vi "Begin.vi"(8 "error in":errorcluster) -> (0 "error out":errorcluster)   [LabVIEW 2019]
doc: "Called before other user functions, this VI is expected to open initial I/O refnums, load in file data, and do all program initialization. Notice that the <B>error out</B> terminal is simply used for data flow. Wiring it to other structures or subVIs ensures that this VI runs first."
uses:
  <vilib>/Rock Robotics/SystemInterfaces/i2clib/i2c_bus.ctl
  <vilib>/Rock Robotics/WPI/DriverStation/WPI_DriverStationRobotMode2.ctl
  <vilib>/Rock Robotics/WPI/Joystick/WPI_JoystickDeviceEnum.ctl
  <vilib>/Rock Robotics/WPI/SafetyOutput/WPI_SafetyOutputConfigMenu.ctl
  <vilib>/Rock Robotics/WPI/ThirdParty/Phoenix-LabVIEW/Motor Controller/Controls/CTRE_Phoenix_MotorControl_ControlMode.ctl
  <vilib>/Rock Robotics/WPI/Solenoid/WPI_SolenoidChannel.ctl
  <vilib>/Rock Robotics/WPI/ThirdParty/Phoenix-LabVIEW/Motor Controller/Controls/CTRE_Phoenix_MotorControl_NeutralMode.ctl
  <vilib>/Rock Robotics/WPI/ThirdParty/Phoenix-LabVIEW/Motor Controller/Controls/CTRE_Phoenix_MotorControl_FeedbackDevice.ctl
  <vilib>/Rock Robotics/WPI/ThirdParty/REV Robotics/SPARK MAX/Typedef/Spark MAX Motor Type.ctl
  <vilib>/Rock Robotics/WPI/ThirdParty/Phoenix-LabVIEW/Motor Controller/Controls/CTRE_Phoenix_MotorControl_FeedbackDevice_TalonFX.ctl
  <vilib>/Rock Robotics/WPI/ThirdParty/Phoenix-LabVIEW/Motor Controller/Controls/CTRE_Phoenix_MotorControl_VelocityMeasurementPeriod.ctl
  <vilib>/Rock Robotics/SystemInterfaces/DIO/FPGA_DIOChannel.ctl
  Robot Global Data.vi
  <vilib>/Rock Robotics/Network Tables/NT Write String Array.vi
  <vilib>/Rock Robotics/WPI/Solenoid/WPI_SolenoidOpenDouble.vi
  <vilib>/Rock Robotics/WPI/RobotDrive/WPI_RobotDriveOpen4MotorWithExistingMotors.vi
panel:
  in  "Blue Calibration":cluster{"R":dbl, "G":dbl, "B":dbl}={"R"=0.143, "G"=0.427, "B"=0.429}
  in  "Green Calibration":cluster{"R":dbl, "G":dbl, "B":dbl}={"R"=0.197, "G"=0.561, "B"=0.24}
  in  "Red Calibration":cluster{"R":dbl, "G":dbl, "B":dbl}={"R"=0.561, "G"=0.323, "B"=0.114}
  in  "Yellow Calibration":cluster{"R":dbl, "G":dbl, "B":dbl}={"R"=0.361, "G"=0.524, "B"=0.113}
  in  "I2C Bus":T1
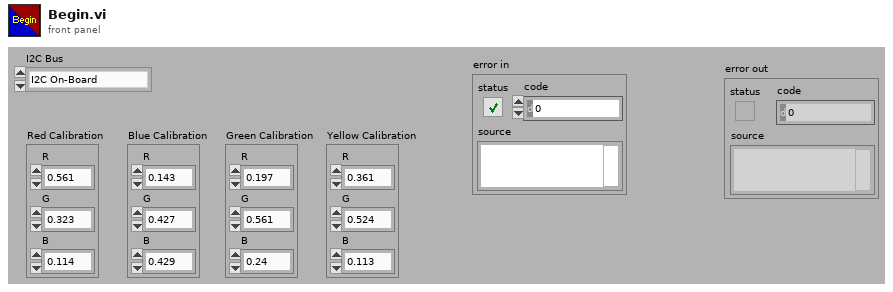
[diagram p1: front panel]
types:
  T1 = typedef "i2c_bus.ctl" = enum16{"I2C On-Board", "I2C MXP", "Invalid"}
  T2 = typedef "CTRE_Phoenix_MotorControl_NeutralMode.ctl" = enum8{"EEPROMSetting", "Override to Coast", "Override to Brake"}
  T3 = typedef "WPI_SolenoidChannel.ctl" = enum8{"Solenoid 0", "Solenoid 1", "Solenoid 2", "Solenoid 3", "Solenoid 4", "Solenoid 5", "Solenoid 6", "Solenoid 7", "Invalid"}
  T4 = typedef "FPGA_DIOChannel.ctl" = enum8{"DIO 0", "DIO 1", "DIO 2", "DIO 3", "DIO 4", "DIO 5", "DIO 6", "DIO 7", "DIO 8", "DIO 9", "DIO MXP 0", "DIO MXP 1", "DIO MXP 2", "DIO MXP 3", "DIO MXP 4", "DIO MXP 5", "DIO MXP 6", "DIO MXP 7", "DIO MXP 8", "DIO MXP 9", "DIO MXP 10", "DIO MXP 11", "DIO MXP 12", "DIO MXP 13", "DIO MXP 14", "DIO MXP 15", "SPI Port CS1", "SPI Port CS2", "SPI Port CS3", "SPI Port MISO", "SPI Port MOSI", "Invalid"}
  T5 = typedef "CTRE_Phoenix_MotorControl_VelocityMeasurementPeriod.ctl" = u16
  T6 = typedef "CTRE_Phoenix_MotorControl_FeedbackDevice_TalonFX.ctl" = i8
  T7 = typedef "CTRE_Phoenix_MotorControl_ControlMode.ctl" = u16
  T8 = typedef "Spark MAX Motor Type.ctl" = enum16{"Brushed", "Brushless"}
  T9 = typedef "CTRE_Phoenix_MotorControl_FeedbackDevice.ctl" = i8
  T10 = typedef "WPI_SafetyOutputConfigMenu.ctl" = enum16{"Enable", "Disable"}
  T11 = typedef "WPI_JoystickDeviceEnum.ctl" = enum16{"USB 0", "USB 1", "USB 2", "USB 3", "USB 4", "USB 5"}
  T12 = typedef "WPI_DriverStationRobotMode2.ctl" = enum16{"Autonomous Disabled", "Autonomous Enabled", "Teleop Disabled", "Teleop Enabled", "Disconnected", "Finish", "Test Disabled", "Test Enabled", "Emergency Stopped"}
  T13 = typedef "Color Sensor V3 DevRef.ctl" = cluster{"I2CDevRef":T14}
  T14 = typedef "WPI_I2CDevRef.ctl" = cluster{"DevStatus":errorcluster, "Device Address":u8, "Handle":i32, "I2C Bus":T1}
  T15 = typedef "WPI_JoystickDevRef.ctl" = cluster{"Device":T11}
  T16 = typedef "WPI_DigitalInputDevRef.ctl" = cluster{"DevStatus":errorcluster, "DIO Channel":T4}
  T17 = typedef "WPI_MotorControlDeviceRef.ctl" = cluster{"DeviceStatus":errorcluster, "Type":T18, "PWM":cluster{"PWM Channel":T19, "DeadBand":T20}, "CAN":cluster{"Device Number":u8, "SetOutput VI Ref":variant, "GetOutput VI Ref":variant, "Enable VI Ref":variant, "Disable VI Ref":variant, "Data":variant}, "Invert":bool, "DIO PWM":cluster{"PWM \"Enable\" Channel":T19, "DIOChannel":T4, "PWM Rate":dbl}}
  T18 = typedef "WPI_MotorControlType.ctl" = enum16{"PWM", "CAN", "DIO PWM"}
  T19 = typedef "FPGA_DIOPWMChannel.ctl" = enum8{"PWM 0", "PWM 1", "PWM 2", "PWM 3", "PWM 4", "PWM 5", "PWM 6", "PWM 7", "PWM 8", "PWM 9", "PWM MXP 0", "PWM MXP 1", "PWM MXP 2", "PWM MXP 3", "PWM MXP 4", "PWM MXP 5", "PWM MXP 6", "PWM MXP 7", "PWM MXP 8", "PWM MXP 9", "Invalid"}
  T20 = typedef "WPI_PWMDeadband.ctl" = cluster{"Name":string, "maxPositivePwm":i32, "minPositivePwm":i32, "centerPwm":i32, "maxNegativePwm":i32, "minNegativePwm":i32, "angularRange":u16}
  T21 = typedef "WPI_SolenoidDevRef.ctl" = cluster{"DevStatus":errorcluster, "Pneumatics Control Module":u8, "Forward Solenoid Channel":T3, "Reverse Solenoid Channel":T3}
  T22 = typedef "WPI_RobotDriveDevRef.ctl" = cluster{"DevStatus":errorcluster, "Motors[]":T17[], "Square Inputs":bool, "Max Output":dbl}
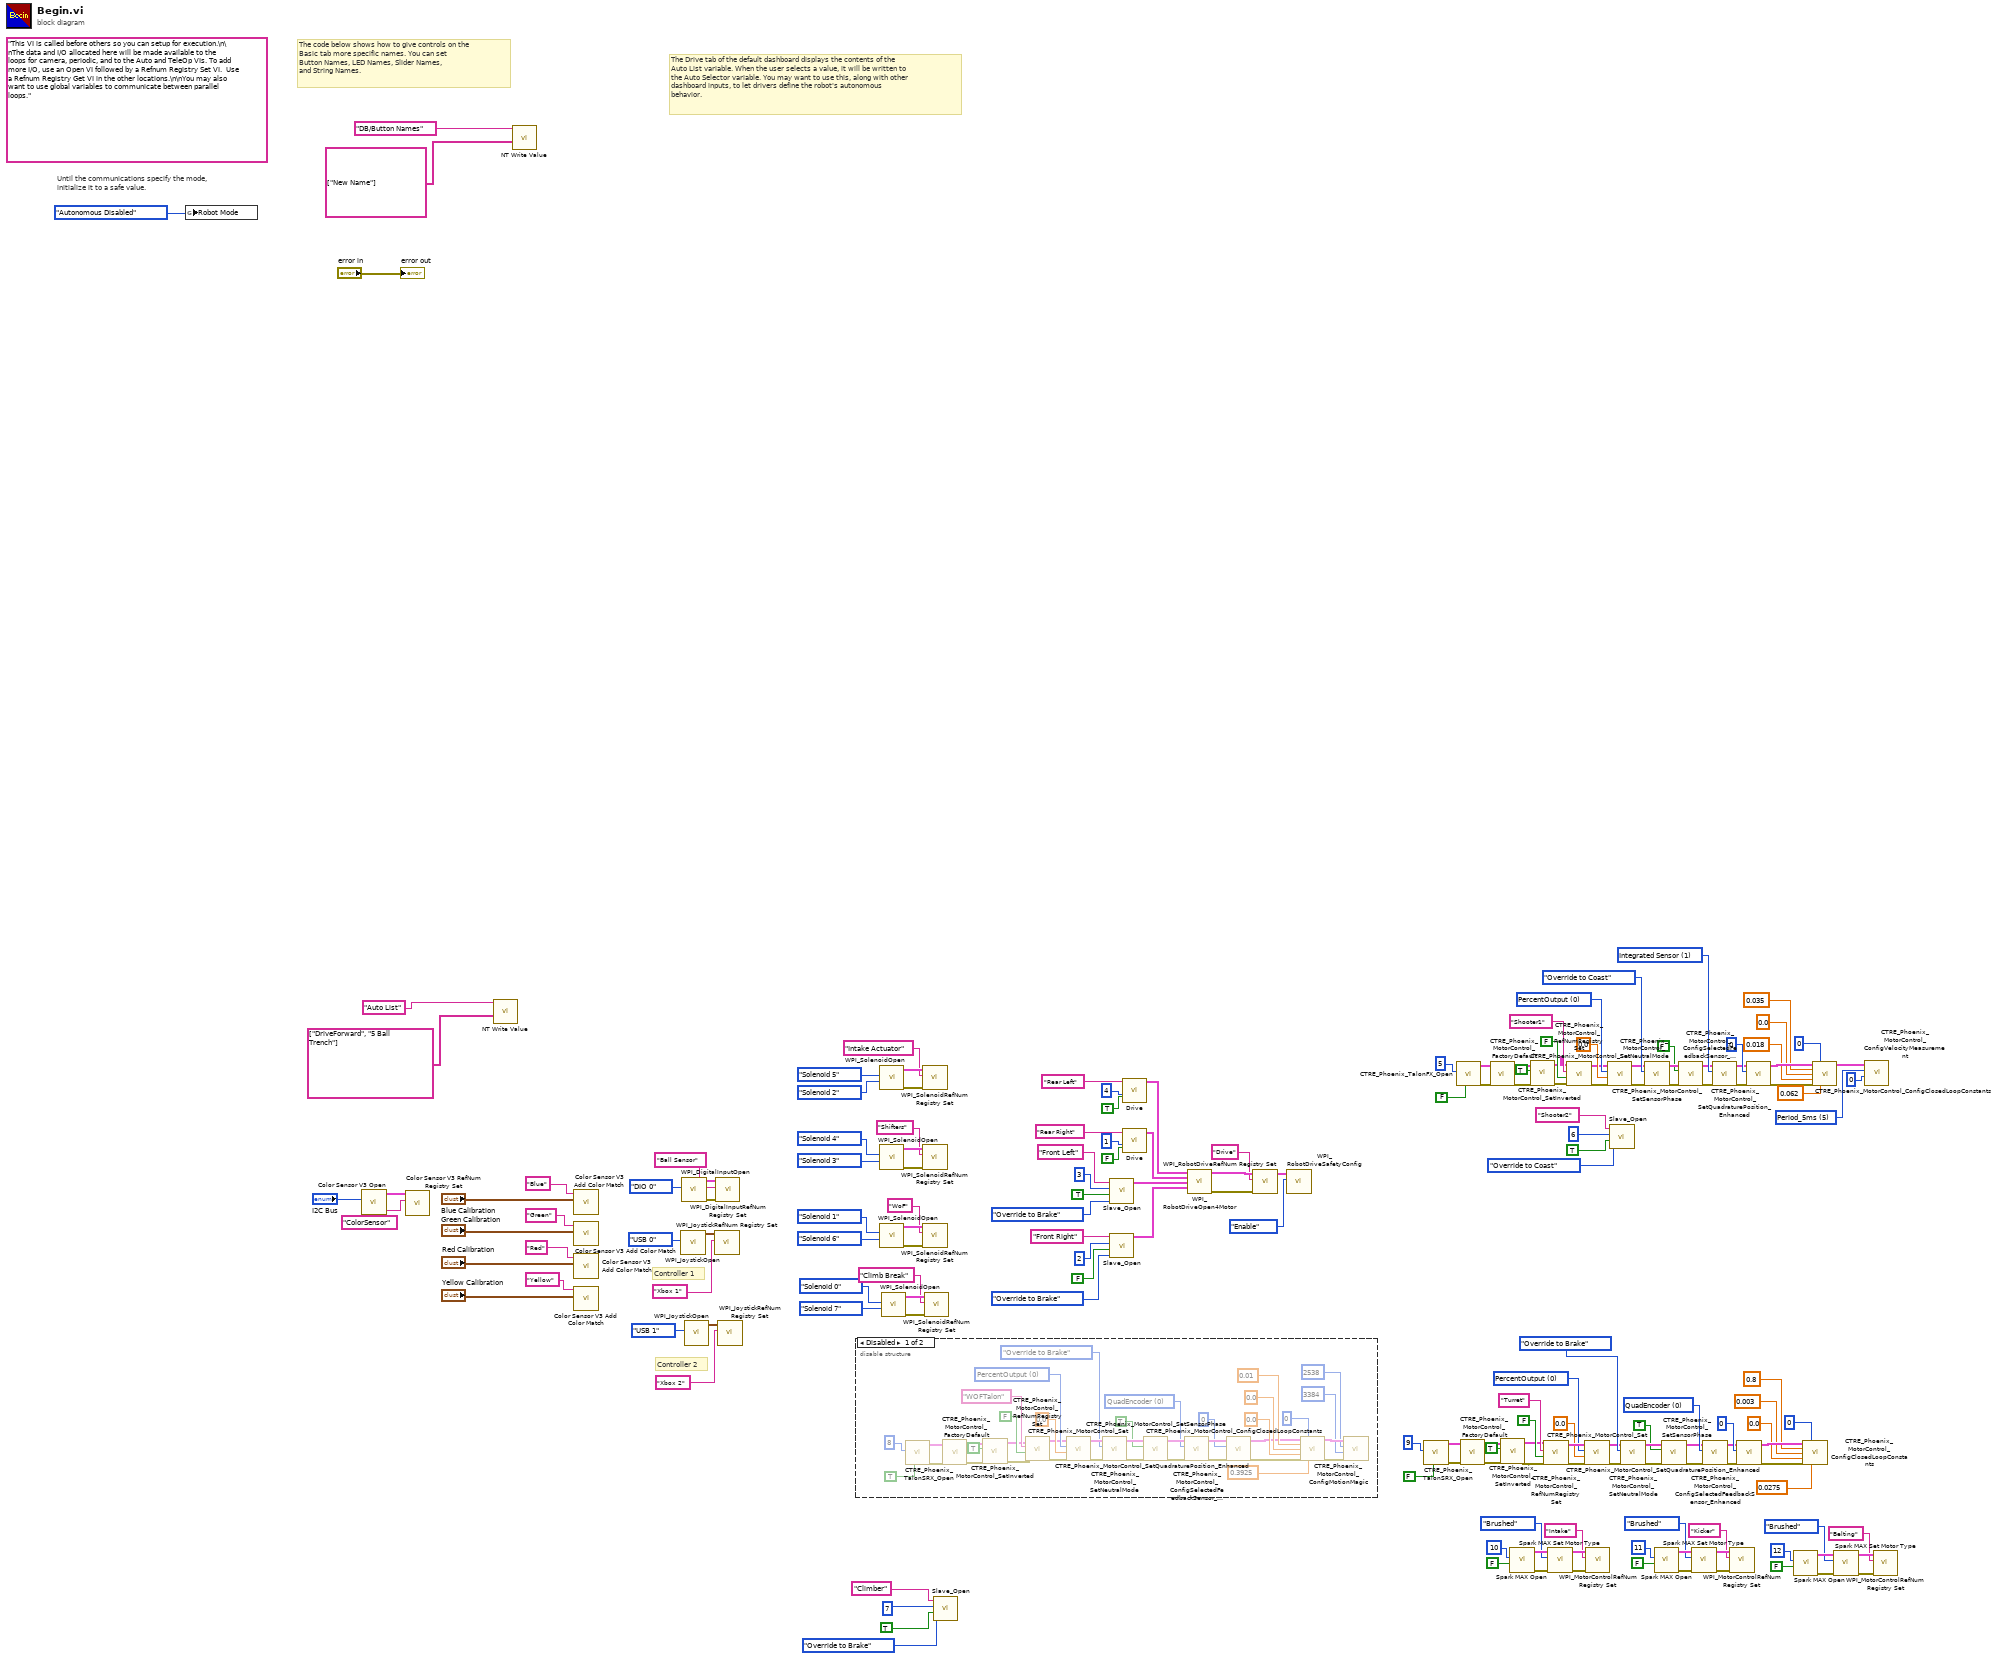
[diagram p0: block diagram]
diagram:
  w88 = T5 5 items=["Period_1ms"=1, "Period_2ms"=2, "Period_5ms"=5, "Period_10ms"=10, "Period_20ms"=20, "Period_25ms"=25, "Period_50ms"=50, "Period_100ms"=100] ("Velocity Measurement Period")
  w78 = T6 1 items=["Integrated Sensor"=1, "Sensor Sum (S0 + S1)"=9, "Sensor Difference (D0 - D1)"=10, "Remote Source 0"=11, "Remote Source 1"=12, "None"=14, "Software Emulated"=15] ("Talon FX Feedback Device")
  w76 = T7 0 items=["PercentOutput"=0, "Position"=1, "Velocity"=2, "Current"=3, "Follower"=5, "MotionProfile"=6, "MotionMagic"=7, "MotionProfileArc"=10, "Disabled"=15] ("Control Mode")
  w131 = T9 0 items=["None"=-1, "QuadEncoder"=0, "Analog"=2, "Tachometer"=4, "Pulse Width Encoded Position"=8, "Sensor Sum (S0 + S1)"=9, "Sensor Difference (D0 - D1)"=10, "Remote Source 0"=11, "Remote Source 1"=12, "Software Emulated"=15] ("Feedback Device")
  w136 = T7 0 items=["PercentOutput"=0, "Position"=1, "Velocity"=2, "Current"=3, "Follower"=5, "MotionProfile"=6, "MotionMagic"=7, "MotionMagicArc"=8, "MotionProfileArc"=10, "Disabled"=15] ("Control Mode")
  (unwired) "This VI is called before others so you can setup for execution.\n\nThe data and I/O allocated here will be made available to the loops for camera, periodic, and to the Auto and TeleOp VIs. To add more I/O, use an Open VI followed by a Refnum Registry Set VI.  Use a Refnum Registry Get VI in the other locations.\n\nYou may also want to use global variables to communicate between parallel loops."
  # "Controller 2"
  # "Controller 1"
  # "The Drive tab of the default dashboard displays the contents of the\nAuto List variable. When the user selects a value, it will be written to\nthe Auto Selector variable. You may want to use this, along with other\ndashboard inputs, to let drivers define the robot's autonomous\nbehavior."
  # "The code below shows how to give controls on the\nBasic tab more specific names. You can set\nButton Names, LED Names, Slider Names,\nand String Names."
  # "Until the communications specify the mode,\ninitialize it to a safe value."
  n1 = global write "Robot Global Data.vi" "Robot Mode"(WPI_DriverStationRobotMode2."Autonomous Disabled" ("Robot Mode")) -> ()
  n2 = call <vilib>:"Color Sensor V3 Open.vi"("I2C Bus"="I2C Bus") -> ("ColorSensorDevRef"=w155:T13)  [unwired: 9 in, 1 out]
  n3 = call <vilib>:"Color Sensor V3 RefNum Registry Set.vi"("refnum name"="ColorSensor", "ColorSensorDevRef"=w155) -> ()  [unwired: 8 in, 2 out]
  n4 = call-poly <vilib>:"NT Write Value.vi"("String Array"=string[] ["DriveForward", "5 Ball Trench"], "Name"="Auto List") -> ()  [unwired: 9 in, 1 out]
  n5 = call-poly <vilib>:"NT Write Value.vi"("String Array"=string[] ["New Name"], "Name"="DB/Button Names") -> ()  [unwired: 9 in, 1 out]
  n6 = call <vilib>:"Color Sensor V3 Add Color Match.vi"("Color"="Blue Calibration", "Name"="Blue") -> ()  [unwired: 10 in]
  n7 = call <vilib>:"Color Sensor V3 Add Color Match.vi"("Color"="Green Calibration", "Name"="Green") -> ()  [unwired: 10 in]
  n8 = call <vilib>:"Color Sensor V3 Add Color Match.vi"("Color"="Red Calibration", "Name"="Red") -> ()  [unwired: 10 in]
  n9 = call <vilib>:"Color Sensor V3 Add Color Match.vi"("Color"="Yellow Calibration", "Name"="Yellow") -> ()  [unwired: 10 in]
  n10 = call <vilib>:"WPI_JoystickOpen.vi"("JoystickDevice"=WPI_JoystickDeviceEnum."USB 0") -> ("JoystickDevRef"=w171:T15)  [unwired: 10 in]
  n11 = call <vilib>:"WPI_DigitalInputOpen.vi"("DIO Channel"=FPGA_DIOChannel."DIO 0") -> ("error out"=w59:errorcluster, "DigitalInputDevRef"=w58:T16)  [unwired: 9 in]
  n12 = call <vilib>:"WPI_JoystickOpen.vi"("JoystickDevice"=WPI_JoystickDeviceEnum."USB 1") -> ("JoystickDevRef"=w152:T15)  [unwired: 10 in]
  n13 = call <vilib>:"WPI_JoystickRefNum Registry Set.vi"("refnum name"="Xbox 1", "JoystickDevRef"=w171) -> ()  [unwired: 8 in, 2 out]
  n14 = call <vilib>:"WPI_DigitalInputRefNum Registry Set.vi"("error in (no error)"=w59, "refnum name"="Ball Sensor", "DigitalInputDevRef"=w58) -> ()  [unwired: 7 in, 2 out]
  n15 = call <vilib>:"WPI_JoystickRefNum Registry Set.vi"("refnum name"="Xbox 2", "JoystickDevRef"=w152) -> ()  [unwired: 8 in, 2 out]
  n16 = disable-structure shown="Disabled" {
    frame Disabled {
      w200 = T9 0 items=["None"=-1, "QuadEncoder"=0, "Analog"=2, "Tachometer"=4, "Pulse Width Encoded Position"=8, "Sensor Sum (S0 + S1)"=9, "Sensor Difference (D0 - D1)"=10, "Remote Source 0"=11, "Remote Source 1"=12, "Software Emulated"=15] ("Feedback Device")
      w195 = T7 0 items=["PercentOutput"=0, "Position"=1, "Velocity"=2, "Current"=3, "Follower"=5, "MotionProfile"=6, "MotionMagic"=7, "MotionMagicArc"=8, "MotionProfileArc"=10, "Disabled"=15] ("Control Mode")
      n17 = call <vilib>:"CTRE_Phoenix_TalonSRX_Open.vi"("Invert"=TRUE, "Device Number"=u8 8) -> ("error out"=w179:errorcluster, "CAN Talon SRX Ref"=w180:T17)  [unwired: 8 in]
      n18 = call <vilib>:"CTRE_Phoenix_MotorControl_FactoryDefault.vi"("error in"=w179, "PhoenixMotorControlDevRef"=w180) -> ("error out"=w178:errorcluster, "PhoenixMotorControlDevRef"=w177:T17)  [unwired: 8 in]
      n19 = call <vilib>:"CTRE_Phoenix_MotorControl_SetInverted.vi"("error in (no error)"=w178, "Invert?"=TRUE, "PhoenixMotorControlDevRef"=w177) -> ("error out"=w174:errorcluster, "PhoenixMotorControlDevRef"=w175:T17)  [unwired: 7 in]
      n20 = call <vilib>:"CTRE_Phoenix_MotorControl_RefNumRegistrySet.vi"("error in (no error)"=w174, "Test Mode Only"=FALSE, "refnum name"="WOFTalon", "PhoenixMotorControlDevRef"=w175) -> ("error out"=w193:errorcluster, "PhoenixMotorControlDevRef"=w194:T17)  [unwired: 6 in]
      n21 = call <vilib>:"CTRE_Phoenix_MotorControl_Set.vi"("error in (no error)"=w193, "Output"=0.0, "Control Mode"=w195, "PhoenixMotorControlDevRef"=w194) -> ("error out"=w204:errorcluster, "PhoenixMotorControlDevRef"=w208:T17)  [unwired: 6 in]
      n22 = call <vilib>:"CTRE_Phoenix_MotorControl_SetNeutralMode.vi"("error in (no error)"=w204, "Motor Control Neutral Mode"=CTRE_Phoenix_MotorControl_NeutralMode."Override to Brake", "PhoenixMotorControlDevRef"=w208) -> ("error out"=w206:errorcluster, "PhoenixMotorControlDevRef"=w205:T17)  [unwired: 7 in]
      n23 = call <vilib>:"CTRE_Phoenix_MotorControl_SetSensorPhase.vi"("error in (no error)"=w206, "PhaseSensor"=TRUE, "PhoenixMotorControlDevRef"=w205) -> ("error out"=w202:errorcluster, "PhoenixMotorControlDevRef"=w201:T17)  [unwired: 7 in]
      n24 = call <vilib>:"CTRE_Phoenix_MotorControl_ConfigSelectedFeedbackSensor_Enhanced.vi"("error in (no error)"=w202, "Feedback Device"=w200, "PhoenixMotorControlDevRef"=w201) -> ("error out"=w198:errorcluster, "PhoenixMotorControlDevRef"=w199:T17)  [unwired: 7 in]
      n25 = call <vilib>:"CTRE_Phoenix_MotorControl_SetQuadraturePosition_Enhanced.vi"("error in (no error)"=w198, "New Position"=0, "PhoenixMotorControlDevRef"=w199) -> ("error out"=w181:errorcluster, "PhoenixMotorControlDevRef"=w182:T17)  [unwired: 7 in]
      n26 = call <vilib>:"CTRE_Phoenix_MotorControl_ConfigClosedLoopConstants.vi"("PhoenixMotorControlDevRef"=w182, "slotIdx"=0, "P"=0.01, "I"=0.0, "D"=0.0, "error in (no error)"=w181, "F"=0.3925) -> ("PhoenixMotorControlDevRef"=w190:T17, "error out"=w191:errorcluster)  [unwired: 7 in]
      n27 = call <vilib>:"CTRE_Phoenix_MotorControl_ConfigMotionMagic.vi"("error in (no error)"=w191, "Acceleration"=3384, "Cruise Velocity"=2538, "PhoenixMotorControlDevRef"=w190) -> ()  [unwired: 6 in, 2 out]
    }
    frame Enabled {
    }
  }
  n28 = call-poly <vilib>:"WPI_SolenoidOpen.vi"("Reverse Solenoid Channel"=WPI_SolenoidChannel."Solenoid 2", "Forward Solenoid Channel"=WPI_SolenoidChannel."Solenoid 5") -> ("error out"=w46:errorcluster, "SolenoidDevRef"=w45:T21)  [unwired: 8 in]
  n29 = call-poly <vilib>:"WPI_SolenoidOpen.vi"("Reverse Solenoid Channel"=WPI_SolenoidChannel."Solenoid 3", "Forward Solenoid Channel"=WPI_SolenoidChannel."Solenoid 4") -> ("error out"=w117:errorcluster, "SolenoidDevRef"=w116:T21)  [unwired: 8 in]
  n30 = call-poly <vilib>:"WPI_SolenoidOpen.vi"("Reverse Solenoid Channel"=WPI_SolenoidChannel."Solenoid 6", "Forward Solenoid Channel"=WPI_SolenoidChannel."Solenoid 1") -> ("error out"=w55:errorcluster, "SolenoidDevRef"=w54:T21)  [unwired: 8 in]
  n31 = call-poly <vilib>:"WPI_SolenoidOpen.vi"("Reverse Solenoid Channel"=WPI_SolenoidChannel."Solenoid 7", "Forward Solenoid Channel"=WPI_SolenoidChannel."Solenoid 0") -> ("error out"=w51:errorcluster, "SolenoidDevRef"=w50:T21)  [unwired: 8 in]
  n32 = call <vilib>:"WPI_SolenoidRefNum Registry Set.vi"("error in (no error)"=w46, "refnum name"="Intake Actuator", "SolenoidDevRef"=w45) -> ()  [unwired: 7 in, 2 out]
  n33 = call <vilib>:"WPI_SolenoidRefNum Registry Set.vi"("error in (no error)"=w117, "refnum name"="Shifters", "SolenoidDevRef"=w116) -> ()  [unwired: 7 in, 2 out]
  n34 = call <vilib>:"WPI_SolenoidRefNum Registry Set.vi"("error in (no error)"=w55, "refnum name"="WoF", "SolenoidDevRef"=w54) -> ()  [unwired: 7 in, 2 out]
  n35 = call <vilib>:"WPI_SolenoidRefNum Registry Set.vi"("error in (no error)"=w51, "refnum name"="Climb Break", "SolenoidDevRef"=w50) -> ()  [unwired: 7 in, 2 out]
  n36 = call "Slave_Open.vi"("Motor Control Neutral Mode"=CTRE_Phoenix_MotorControl_NeutralMode."Override to Brake", "Invert"=TRUE, "Device Number"=u8 7, "Motor Name"="Climber" ("refnum name")) -> ()  [unwired: 7 in, 1 out]
  n37 = call "Slave_Open.vi"("Motor Control Neutral Mode"=CTRE_Phoenix_MotorControl_NeutralMode."Override to Brake", "Invert"=TRUE, "Device Number"=u8 3, "Motor Name"="Front Left" ("refnum name")) -> ("PhoenixMotorControlDevRef"=w12:T17)  [unwired: 7 in]
  n38 = call "Slave_Open.vi"("Motor Control Neutral Mode"=CTRE_Phoenix_MotorControl_NeutralMode."Override to Brake", "Invert"=FALSE, "Device Number"=u8 2, "Motor Name"="Front Right" ("refnum name")) -> ("PhoenixMotorControlDevRef"=w11:T17)  [unwired: 7 in]
  n39 = call "Drive.vi"("Invert"=TRUE, "Device Number"=u8 4, "Motor Name"="Rear Left" ("refnum name")) -> ("Motor Out"=w118:T17)  [unwired: 8 in]
  n40 = call "Drive.vi"("Invert"=FALSE, "Device Number"=u8 1, "Motor Name"="Rear Right" ("refnum name")) -> ("Motor Out"=w33:T17)  [unwired: 8 in]
  n41 = call-poly <vilib>:"WPI_RobotDriveOpen4Motor.vi"("Rear Left Motor Dev Ref"=w118, "Rear Right Motor Dev Ref"=w33, "Front Left Motor Dev Ref"=w12, "Front Right Motor Dev Ref"=w11) -> ("RobotDriveDevRef"=w150:T22, "error out"=w148:errorcluster)  [unwired: 10 in]
  n42 = call <vilib>:"WPI_RobotDriveRefNum Registry Set.vi"("error in (no error)"=w148, "refnum name"="Drive", "RobotDriveDevRef"=w150) -> ("RobotDriveDevRef"=w147:T22)  [unwired: 1 in, 7 out]
  n43 = call <vilib>:"WPI_RobotDriveSafetyConfig.vi"("mode"=WPI_SafetyOutputConfigMenu."Enable", "RobotDriveDevRef"=w147) -> ()  [unwired: 8 in, 2 out]
  n44 = call <vilib>:"CTRE_Phoenix_TalonSRX_Open.vi"("Invert"=FALSE, "Device Number"=u8 9) -> ("error out"=w20:errorcluster, "CAN Talon SRX Ref"=w19:T17)  [unwired: 8 in]
  n45 = call <vilib>:"CTRE_Phoenix_TalonFX_Open.vi"("Invert"=FALSE, "Device Number"=u8 5) -> ("error out"=w27:errorcluster, "CAN Talon SRX Ref"=w26:T17)  [unwired: 8 in]
  n46 = call <vilib>:"CTRE_Phoenix_MotorControl_FactoryDefault.vi"("error in"=w20, "PhoenixMotorControlDevRef"=w19) -> ("error out"=w25:errorcluster, "PhoenixMotorControlDevRef"=w24:T17)  [unwired: 8 in]
  n47 = call <vilib>:"CTRE_Phoenix_MotorControl_FactoryDefault.vi"("error in"=w27, "PhoenixMotorControlDevRef"=w26) -> ("error out"=w32:errorcluster, "PhoenixMotorControlDevRef"=w31:T17)  [unwired: 8 in]
  n48 = call <vilib>:"CTRE_Phoenix_MotorControl_SetInverted.vi"("error in (no error)"=w25, "Invert?"=TRUE, "PhoenixMotorControlDevRef"=w24) -> ("error out"=w21:errorcluster, "PhoenixMotorControlDevRef"=w22:T17)  [unwired: 7 in]
  n49 = call <vilib>:"Spark MAX Open.vi"("Invert"=FALSE, "Device Number"=u8 10) -> ("error out"=w112:errorcluster, "MotorControlDeviceRef"=w113:T17)  [unwired: 8 in]
  n50 = call <vilib>:"CTRE_Phoenix_MotorControl_SetInverted.vi"("error in (no error)"=w32, "Invert?"=TRUE, "PhoenixMotorControlDevRef"=w31) -> ("error out"=w28:errorcluster, "PhoenixMotorControlDevRef"=w29:T17)  [unwired: 7 in]
  n51 = call <vilib>:"CTRE_Phoenix_MotorControl_RefNumRegistrySet.vi"("error in (no error)"=w21, "Test Mode Only"=FALSE, "refnum name"="Turret", "PhoenixMotorControlDevRef"=w22) -> ("error out"=w138:errorcluster, "PhoenixMotorControlDevRef"=w137:T17)  [unwired: 6 in]
  n52 = call <vilib>:"Spark MAX Set Motor Type.vi"("error in (no error)"=w112, "Motor Type"=Spark_MAX_Motor_Type."Brushed", "MotorControlDevRef"=w113) -> ("error out"=w110:errorcluster, "MotorControlDeviceRef"=w109:T17)  [unwired: 7 in]
  n53 = call <vilib>:"CTRE_Phoenix_MotorControl_RefNumRegistrySet.vi"("error in (no error)"=w28, "Test Mode Only"=FALSE, "refnum name"="Shooter1", "PhoenixMotorControlDevRef"=w29) -> ("error out"=w65:errorcluster, "PhoenixMotorControlDevRef"=w66:T17)  [unwired: 6 in]
  n54 = call <vilib>:"CTRE_Phoenix_MotorControl_Set.vi"("error in (no error)"=w138, "Output"=0.0, "Control Mode"=w136, "PhoenixMotorControlDevRef"=w137) -> ("error out"=w128:errorcluster, "PhoenixMotorControlDevRef"=w124:T17)  [unwired: 6 in]
  n55 = call <vilib>:"WPI_MotorControlRefNum Registry Set.vi"("error in (no error)"=w110, "refnum name"="Intake", "MotorControlDevRef"=w109) -> ()  [unwired: 7 in, 2 out]
  n56 = call <vilib>:"CTRE_Phoenix_MotorControl_Set.vi"("error in (no error)"=w65, "Output"=0.0, "Control Mode"=w76, "PhoenixMotorControlDevRef"=w66) -> ("error out"=w67:errorcluster, "PhoenixMotorControlDevRef"=w68:T17)  [unwired: 6 in]
  n57 = call "Slave_Open.vi"("Motor Control Neutral Mode"=CTRE_Phoenix_MotorControl_NeutralMode."Override to Coast", "Invert"=TRUE, "Device Number"=u8 6, "Motor Name"="Shooter2" ("refnum name")) -> ()  [unwired: 7 in, 1 out]
  n58 = call <vilib>:"CTRE_Phoenix_MotorControl_SetNeutralMode.vi"("error in (no error)"=w128, "Motor Control Neutral Mode"=CTRE_Phoenix_MotorControl_NeutralMode."Override to Brake", "PhoenixMotorControlDevRef"=w124) -> ("error out"=w126:errorcluster, "PhoenixMotorControlDevRef"=w127:T17)  [unwired: 7 in]
  n59 = call <vilib>:"CTRE_Phoenix_MotorControl_SetNeutralMode.vi"("error in (no error)"=w67, "Motor Control Neutral Mode"=CTRE_Phoenix_MotorControl_NeutralMode."Override to Coast", "PhoenixMotorControlDevRef"=w68) -> ("error out"=w69:errorcluster, "PhoenixMotorControlDevRef"=w70:T17)  [unwired: 7 in]
  n60 = call <vilib>:"Spark MAX Open.vi"("Invert"=FALSE, "Device Number"=u8 11) -> ("error out"=w96:errorcluster, "MotorControlDeviceRef"=w97:T17)  [unwired: 8 in]
  n61 = call <vilib>:"CTRE_Phoenix_MotorControl_SetSensorPhase.vi"("error in (no error)"=w126, "PhaseSensor"=TRUE, "PhoenixMotorControlDevRef"=w127) -> ("error out"=w129:errorcluster, "PhoenixMotorControlDevRef"=w130:T17)  [unwired: 7 in]
  n62 = call <vilib>:"CTRE_Phoenix_MotorControl_SetSensorPhase.vi"("error in (no error)"=w69, "PhaseSensor"=FALSE, "PhoenixMotorControlDevRef"=w70) -> ("error out"=w71:errorcluster, "PhoenixMotorControlDevRef"=w72:T17)  [unwired: 7 in]
  n63 = call <vilib>:"Spark MAX Set Motor Type.vi"("error in (no error)"=w96, "Motor Type"=Spark_MAX_Motor_Type."Brushed", "MotorControlDevRef"=w97) -> ("error out"=w94:errorcluster, "MotorControlDeviceRef"=w93:T17)  [unwired: 7 in]
  n64 = call <vilib>:"CTRE_Phoenix_MotorControl_ConfigSelectedFeedbackSensor_Enhanced.vi"("error in (no error)"=w129, "Feedback Device"=w131, "PhoenixMotorControlDevRef"=w130) -> ("error out"=w133:errorcluster, "PhoenixMotorControlDevRef"=w132:T17)  [unwired: 7 in]
  n65 = call <vilib>:"CTRE_Phoenix_MotorControl_ConfigSelectedFeedbackSensor_TalonFX.vi"("error in (no error)"=w71, "Talon FX Feedback Device"=w78, "PhoenixMotorControlDevRef"=w72) -> ("error out"=w73:errorcluster, "PhoenixMotorControlDevRef"=w74:T17)  [unwired: 7 in]
  n66 = call <vilib>:"WPI_MotorControlRefNum Registry Set.vi"("error in (no error)"=w94, "refnum name"="Kicker", "MotorControlDevRef"=w93) -> ()  [unwired: 7 in, 2 out]
  n67 = call <vilib>:"CTRE_Phoenix_MotorControl_SetQuadraturePosition_Enhanced.vi"("error in (no error)"=w133, "New Position"=0, "PhoenixMotorControlDevRef"=w132) -> ("error out"=w145:errorcluster, "PhoenixMotorControlDevRef"=w144:T17)  [unwired: 7 in]
  n68 = call <vilib>:"CTRE_Phoenix_MotorControl_SetQuadraturePosition_Enhanced.vi"("error in (no error)"=w73, "New Position"=0, "PhoenixMotorControlDevRef"=w74) -> ("error out"=w87:errorcluster, "PhoenixMotorControlDevRef"=w86:T17)  [unwired: 7 in]
  n69 = call <vilib>:"Spark MAX Open.vi"("Invert"=FALSE, "Device Number"=u8 12) -> ("error out"=w104:errorcluster, "MotorControlDeviceRef"=w105:T17)  [unwired: 8 in]
  n70 = call <vilib>:"CTRE_Phoenix_MotorControl_ConfigClosedLoopConstants.vi"("PhoenixMotorControlDevRef"=w144, "slotIdx"=0, "P"=0.8, "I"=0.003, "D"=0.0, "error in (no error)"=w145, "F"=0.0275) -> ()  [unwired: 7 in, 2 out]
  n71 = call <vilib>:"CTRE_Phoenix_MotorControl_ConfigClosedLoopConstants.vi"("PhoenixMotorControlDevRef"=w86, "slotIdx"=0, "P"=0.035, "I"=0.0, "D"=0.018, "error in (no error)"=w87, "F"=0.062) -> ("PhoenixMotorControlDevRef"=w89:T17)  [unwired: 7 in, 1 out]
  n72 = call <vilib>:"Spark MAX Set Motor Type.vi"("error in (no error)"=w104, "Motor Type"=Spark_MAX_Motor_Type."Brushed", "MotorControlDevRef"=w105) -> ("error out"=w102:errorcluster, "MotorControlDeviceRef"=w101:T17)  [unwired: 7 in]
  n73 = call <vilib>:"CTRE_Phoenix_MotorControl_ConfigVelocityMeasurement.vi"("Window Size"=0, "Velocity Measurement Period"=w88, "PhoenixMotorControlDevRef"=w89) -> ()  [unwired: 7 in, 2 out]
  n74 = call <vilib>:"WPI_MotorControlRefNum Registry Set.vi"("error in (no error)"=w102, "refnum name"="Belting", "MotorControlDevRef"=w101) -> ()  [unwired: 7 in, 2 out]
  "error out" <- "error in"
